vi "CODMn通讯.vi"() -> ()   [LabVIEW 2016, in "斯坦道CODMn.lvlib"]
uses:
  <vilib>/NI/Modbus Library/API/Wrapper/Create TCP Slave.vi
  <vilib>/NI/Modbus Library/API/slave/Modbus Slave.lvclass
  <vilib>/Plasmionique/MB Master/MB_Master/MB_Master.lvclass
  <vilib>/Plasmionique/MB Master/MB Master.lvlib
  <vilib>/Utility/config.llb/NI_LVConfig.lvlib
  <vilib>/NI/Modbus Library/API/Wrapper/API Main.lvlib
panel:
  in  "读取数据":bool
  in  "释放串口":bool
  in  "打开串口":bool
  out "队列中元素数量":i32
  out "元素":cluster{"命令":string}[](array[cluster])
  out "待处理插入数量":i32
  out "读取公式":u16[](array[numeric])
  out "读取参数":u16[](array[numeric])
  out "数据存储":u16[](array[numeric])
  out "温度":bool[](array[boolean])
  out "M输出点":bool[](array[boolean])
  out "ORP、时间":u16[](array[numeric])
  out "测量状态":u16[](array[numeric])
  out "通讯状态":bool
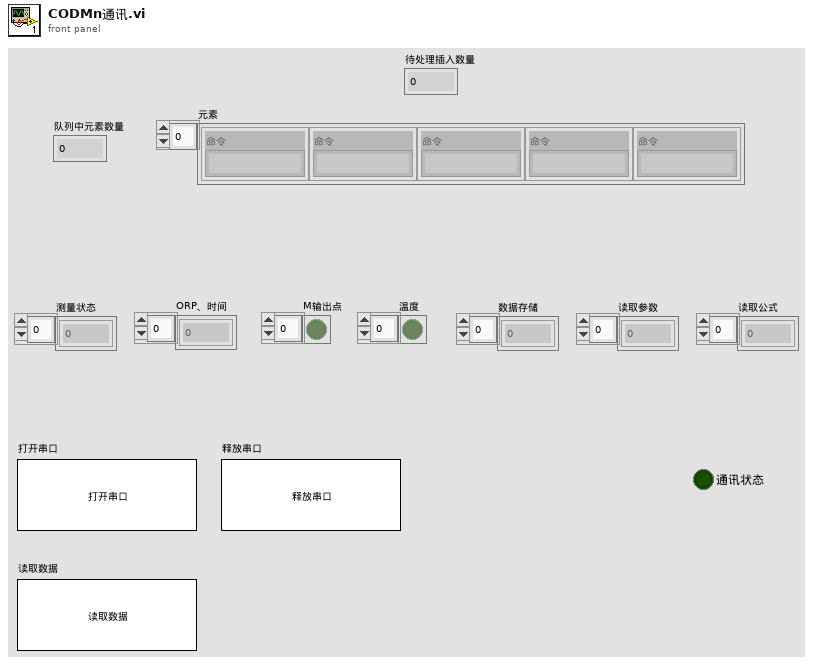
[diagram p1: front panel]
types:
  T1 = cluster{"测量模式":enum16{"水样测量", "标样核查", "零点核查", "跨度核查", "空白测试", "加标回收", "平行样", "校零", "校标"}}
  T2 = cluster{"命令":string, "测量模式":enum16{"水样测量", "标样核查", "零点核查", "跨度核查", "空白测试", "加标回收", "平行样", "校零", "校标"}, "CODMn量程切换":enum32{"H", "L", "AUTO"}}
  T3 = typedef "NI_LVConfig.lvlib/Config Data RefNum.ctl" = refnum<k1>
  T4 = enum16{"空闲", "水样测试", "标样核查", "零点核查", "跨度核查", "空白测试", "平行样测试", "质控样", "空白校准", "标样校准", "加标回收"}
  T5 = enum16{"水样测量", "标样核查", "零点核查", "跨度核查", "空白测试", "加标回收", "平行样", "校零", "校标"}
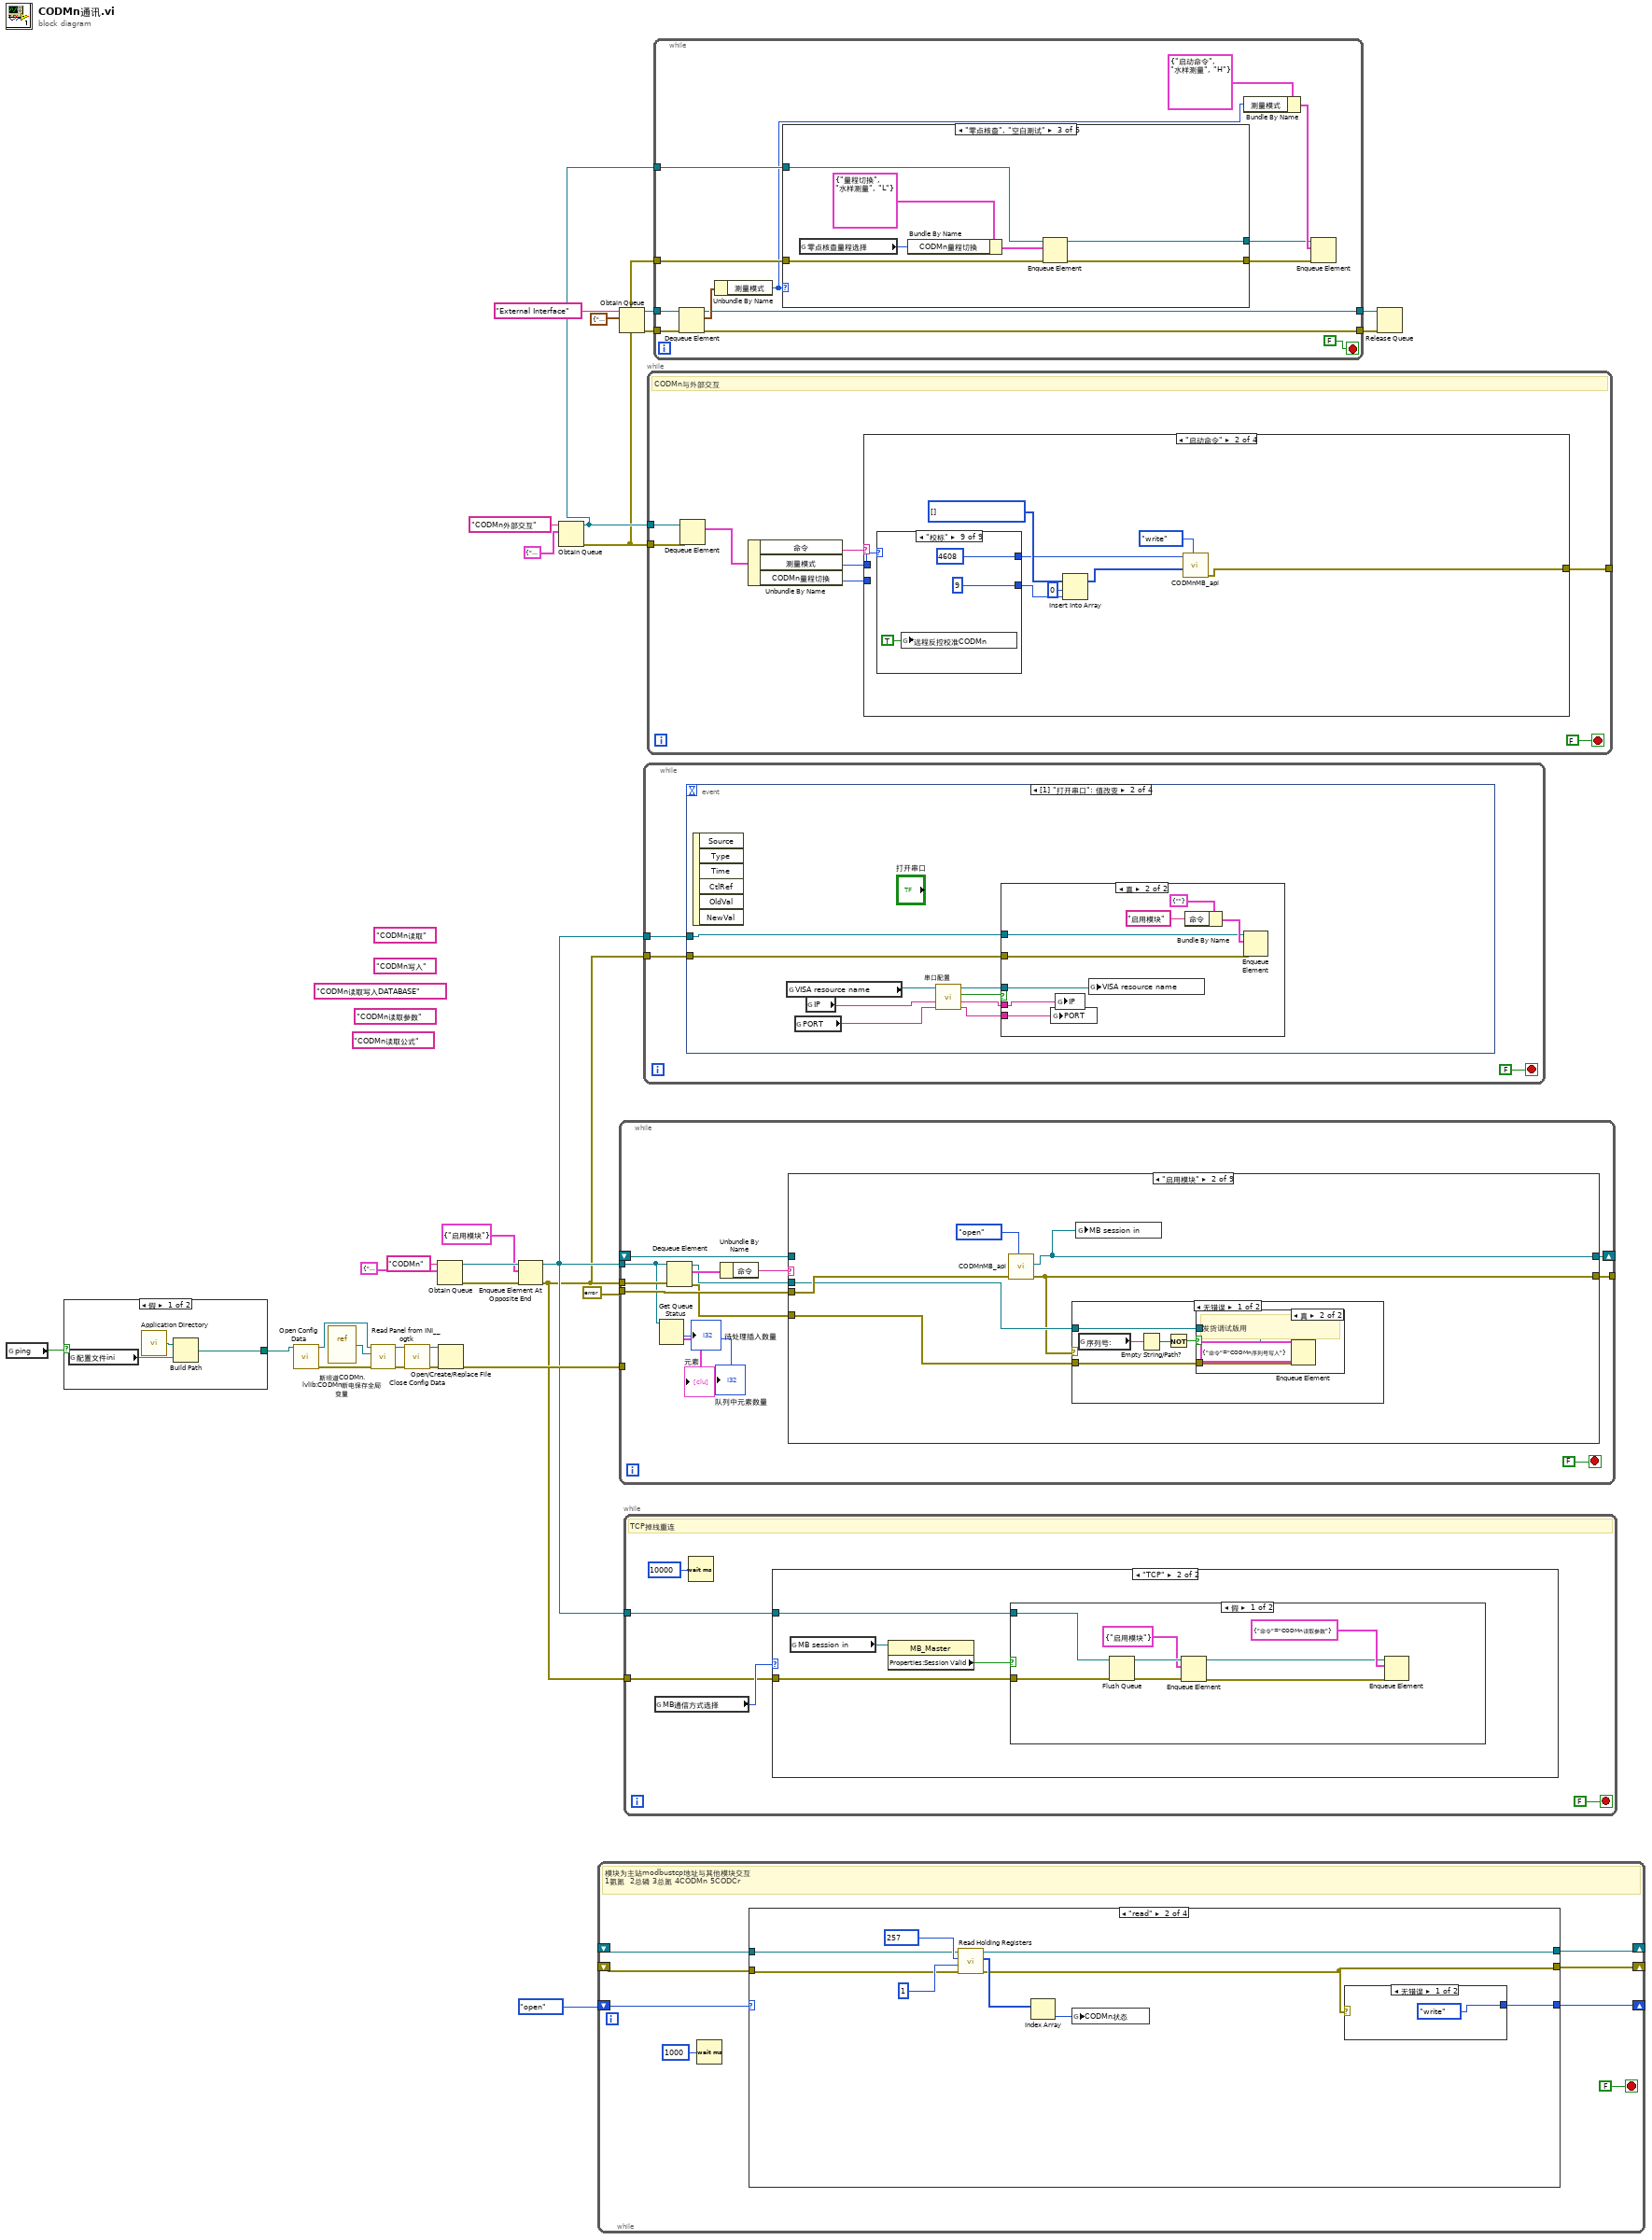
[diagram p0: block diagram]
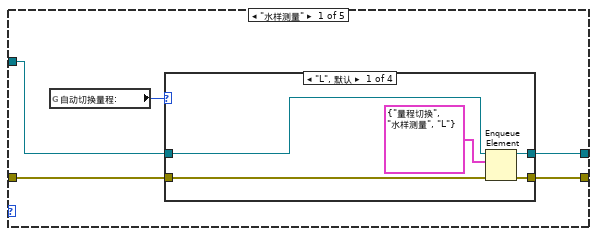
[diagram p2: hidden frame]
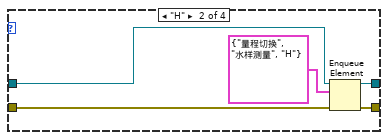
[diagram p3: hidden frame]
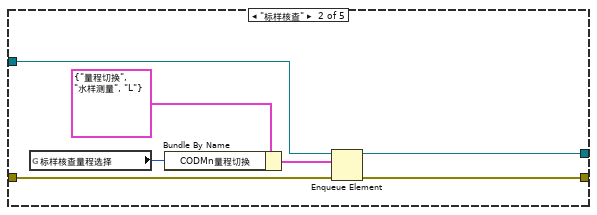
[diagram p6: hidden frame]
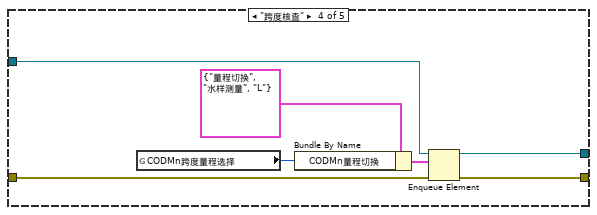
[diagram p7: hidden frame]
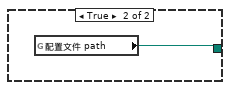
[diagram p9: hidden frame]
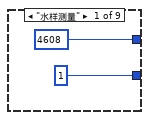
[diagram p11: hidden frame]
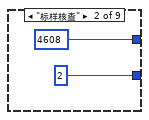
[diagram p12: hidden frame]
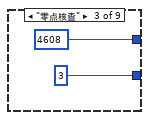
[diagram p13: hidden frame]
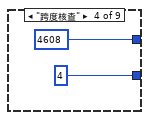
[diagram p14: hidden frame]
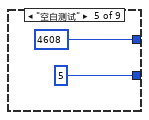
[diagram p15: hidden frame]
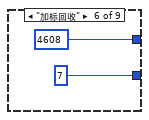
[diagram p16: hidden frame]
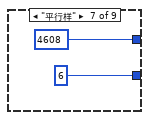
[diagram p17: hidden frame]
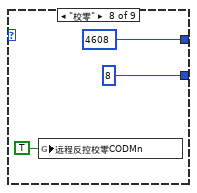
[diagram p18: hidden frame]
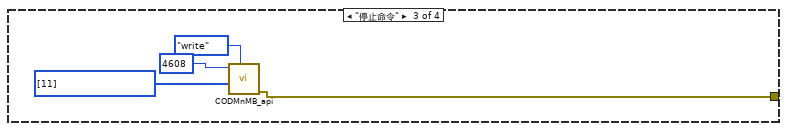
[diagram p19: hidden frame]
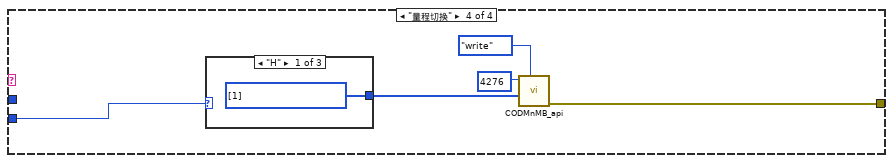
[diagram p20: hidden frame]
diagram:
  (unwired) "CODMn读取公式" ("名称（未命名）")
  (unwired) "CODMn读取写入DATABASE" ("名称（未命名）")
  (unwired) "CODMn读取参数" ("名称（未命名）")
  (unwired) "CODMn读取" ("名称（未命名）")
  (unwired) "CODMn写入" ("名称（未命名）")
  n1 = global read "CODMN外部API.vi" "ping"() -> (w10:bool)
  n2 = case shown="假" w10 {
    tunnel: [w30 w33] -> w9
    frame False {
      n3 = global read "COD内部交互全局.vi" "配置文件ini"() -> (w32:string)
      n4 = call <vilib>:"Application Directory.vi"() -> ("Application Directory"=w31:path)
      n5 = Build Path(base path=w31, name or relative path=w32) -> (appended path=w30:path)
    }
    frame True {
      n6 = global read "CODMN外部API.vi" "配置文件 path"() -> (w33:path)
    }
  }
  n7 = call <vilib>:"Open Config Data.vi"("configuration file path"=w9) -> ("error out"=w20:errorcluster, "refnum"=w23:T3)  [unwired: 8 in, 1 out]
  n8 = vi-ref "斯坦道CODMn.lvlib:CODMn断电保存全局变量.vi"() -> (w22:refnum<vi>)
  n9 = call <userlib>:"Read Panel from INI__ogtk.vi"("error in (no error)"=w20, "VI ref"=w22, "refnum"=w23) -> ("error out"=w19:errorcluster, "refnum out"=w21:T3)  [unwired: 7 in]
  n10 = call <vilib>:"Close Config Data.vi"("error in (no error)"=w19, "refnum"=w21) -> ("error out"=w18:errorcluster, "file path"=w17:path)  [unwired: 8 in]
  n11 = Obtain Queue(name (unnamed)="CODMn" ("名称（未命名）"), element data type=cluster{"命令":string} {"命令"="启用模块"} ("元素")) -> (queue out=w26:refnum<queue>, error out=w25:errorcluster)  [unwired: 3 in, 1 out]
  n12 = Open/Create/Replace File(file path (use dialog)=w17, error in=w18) -> (error out=w16:errorcluster)  [unwired: 4 in, 2 out]
  n13 = Enqueue Element At Opposite End(queue=w26, element=cluster{"命令":string} {"命令"="启用模块"} ("元素"), error in (no error)=w25) -> (queue out=w14:refnum<queue>, error out=w13:errorcluster)  [unwired: 1 in, 1 out]
  n14 = Obtain Queue(name (unnamed)="CODMn外部交互" ("名称（未命名）"), element data type=T2 {"命令"="启动命令", "测量模式"=enum."水样测量", "CODMn量程切换"=enum."AUTO"} ("元素")) -> (queue out=w4:refnum<queue>, error out=w3:errorcluster)  [unwired: 3 in, 1 out]
  n15 = while {
    shift-right: [w39] -> _
    shift-left: _ -> [w41]
    shift-right: [w38] -> _
    shift-left: _ -> [w40]
    shift-right: [w35] -> _
    shift-left: enum16{"open", "read", "write", "close"}."open" -> [w36]
    stop <- FALSE stop-if-true
    # "模块为主站modbustcp地址与其他模块交互\n1氨氮  2总磷 3总氮 4CODMn 5CODCr"
    n16 = Wait (ms)(milliseconds to wait=u32 1000 ("等待时间（毫秒）")) -> ()  [unwired: 1 out]
    n17 = case shown="\"read\"" w36 {
      selector: w36 -> [w50 _ _ _]
      tunnel: w41 -> [w44 w58 w81 w87]
      tunnel: w40 -> [w43 w57 w78 w86]
      tunnel: [w47 w53 w80 w87] -> w39
      tunnel: [w46 w54 w79 w89] -> w38
      tunnel: [w49 w61 w82 enum16{"open", "read", "write", "close"}."open"] -> w35
      frame "open", Default {
        n18 = call-dynamic "Shutdown.vi"("error in"=w43, "Modbus slave in"=w44) -> ("error out"=w42:errorcluster)  [unwired: 9 in]
        n19 = call <vilib>:"Clear Errors.vi"("error in (no error)"=w42) -> ("error out"=w45:errorcluster)  [unwired: 5 in, 1 out]
        n20 = call-poly <vilib>:"Create Modbus Instance.vi"("error in"=w45, "port (502)"=u16 4) -> ("error out"=w46:errorcluster, "TCP slave instance"=w47:refnum<class "Modbus Slave.lvclass">)  [unwired: 8 in]
        n21 = case shown="错误" w46 {
          tunnel: w50 -> [_ w52]
          tunnel: [enum16{"open", "read", "write", "close"}."write" w52] -> w49
          frame No Error {
          }
          frame Error {
          }
        }
      }
      frame "read" {
        n22 = call-dynamic <vilib>:"Read Holding Registers.vi"("error in"=w57, "number of inputs"=u16 1, "starting address"=u16 257, "Modbus slave in"=w58) -> ("error out"=w54:errorcluster, "register values"=w56:u16[], "Modbus slave out"=w53:refnum<class "Modbus Slave.lvclass">)  [unwired: 5 in]
        n23 = Index Array(array=w56) -> (element=w55:u16)  [unwired: 1 in]
        n24 = global write "CODMN外部API.vi" "CODMn状态"(w55) -> ()
        n25 = case shown="无错误" w54 {
          tunnel: [enum16{"open", "read", "write", "close"}."write" enum16{"open", "read", "write", "close"}."close"] -> w61
          frame No Error {
          }
          frame Error {
          }
        }
      }
      frame "write" {
        n26 = global read "COD测量模式全局.vi" "CODMn工作状态"() -> (w68:T4)
        n27 = global read "COD浓度全局变量.vi" "COD浓度（mg/L)"() -> (w70:dbl)
        n28 = global read "COD测量模式全局.vi" "加标回收启动时间"() -> (w73:timestamp)
        n29 = global read "COD测量模式全局.vi" "水样启动时间"() -> (w75:timestamp)
        n30 = global read "运行时序全局变量.vi" "多列列表框"() -> (w72:i32)
        n31 = Build Array(w75) -> (w74:timestamp[])
        n32 = Build Array(w70) -> (w69:dbl[])
        n33 = Build Array(w73) -> (w66:timestamp[])
        n34 = call "浮点转CDAB整形cod.vi"("浮点数"=w69) -> ("CDAB整形输出"=w71:u16[])  [unwired: 10 in]
        n35 = call "DateToHex.vi"("DATE"=w74) -> ("数组"=w77:u16[])  [unwired: 10 in]
        n36 = call "DateToHex.vi"("DATE"=w66) -> ("数组"=w76:u16[])  [unwired: 10 in]
        n37 = Insert Into Array(array=u16[] [] ("values"), new element #1=w68, new element #2=w71, new element #3=w72, new element #4=w76, new element #5=w77) -> (w65:u16[])  [unwired: 1 in]
        n38 = call-dynamic "Write Multiple Holding Registers.vi"("error in"=w78, "registers to write"=w65, "starting address"=u16 0, "Modbus slave in"=w81) -> ("error out"=w79:errorcluster, "Modbus slave out"=w80:refnum<class "Modbus Slave.lvclass">)  [unwired: 6 in]
        n39 = case shown="无错误" w79 {
          tunnel: [enum16{"open", "read", "write", "close"}."read" enum16{"open", "read", "write", "close"}."close"] -> w82
          frame No Error {
          }
          frame Error {
          }
        }
      }
      frame "close" {
        n40 = call-dynamic "Shutdown.vi"("error in"=w86, "Modbus slave in"=w87) -> ("error out"=w85:errorcluster)  [unwired: 9 in]
        n41 = call <vilib>:"Clear Errors.vi"("error in (no error)"=w85) -> ("error out"=w89:errorcluster)  [unwired: 5 in, 1 out]
      }
    }
  }
  n42 = while {
    tunnel: w14 -> [w95]
    tunnel: w13 -> [w102]
    tunnel: [w96] -> _
    shift-right: [w99] -> _
    shift-left: _ -> [w98]
    tunnel: errorcluster {"status"=FALSE, "code"=0, "source"=""} ("error out") -> [w97]
    tunnel: w16 -> [_]
    stop <- FALSE stop-if-true
    n43 = Get Queue Status(queue=w95) -> (# pending insert=→"待处理插入数量":i32, # elements in queue=→"队列中元素数量":i32, elements=→"元素":cluster{"命令":string}[])  [unwired: 2 in, 5 out]
    n44 = Dequeue Element(queue=w95, error in (no error)=w102) -> (queue out=w91:refnum<queue>, element=w101:cluster{"命令":string}, error out=w90:errorcluster)  [unwired: 1 in, 1 out]
    n45 = Unbundle By Name(w101) -> ("命令"=w100:string)
    n46 = case shown="\"启用模块\"" w100 {
      tunnel: [w105 w109 w120 w128 w160 w169 w186 w193 w200] -> w99
      tunnel: [w104 w106 w121 w125 w158 w168 w185 w192 w199] -> w96
      tunnel: w98 -> [w105 _ _ w152 w164 w178 w189 w197 w203]
      tunnel: w97 -> [w104 w110 w122 w151 w161 w177 w188 w196 w201]
      tunnel: w91 -> [_ w108 _ _ _ _ _ _ _]
      tunnel: w90 -> [_ w107 _ _ _ _ _ _ _]
      frame Default {
      }
      frame "启用模块" {
        n47 = call "CODMnMB_api.vi"("STEP"=enum16{"open", "read", "write", "close"}."open", "Error in"=w110) -> ("error out"=w106:errorcluster, "MB session out"=w109:refnum<class "MB_Master.lvclass">)  [unwired: 7 in, 1 out]
        n48 = case shown="无错误" w106 {
          tunnel: w108 -> [w116 _]
          tunnel: w107 -> [w115 _]
          frame No Error {
            n49 = global read "COD内部交互全局.vi" "序列号:"() -> (w114:string)
            n50 = Empty String/Path?(string/path=w114) -> (empty?=w113:bool)
            n51 = Not(x=w113) -> (.not. x?=w112:bool)
            n52 = case shown="真" w112 {
              tunnel: w116 -> [_ w119]
              tunnel: w115 -> [_ w118]
              frame False {
              }
              frame True {
                # "发货调试版用"
                n53 = Enqueue Element(queue=w119, element=cluster{"命令":string} {"命令"="CODMn序列号写入"} ("元素"), error in (no error)=w118) -> ()  [unwired: 1 in, 3 out]
              }
            }
          }
          frame Error {
          }
        }
        n54 = global write "COD浓度全局变量.vi" "MB session in"(w109) -> ()
      }
      frame "停用模块" {
        n55 = call "CODMnMB_api.vi"("STEP"=enum16{"open", "read", "write", "close"}."close", "Error in"=w122) -> ("error out"=w121:errorcluster, "MB session out"=w120:refnum<class "MB_Master.lvclass">)  [unwired: 7 in, 1 out]
      }
      frame "CODMn读取" {
        n56 = call <vilib>:"Read Holding Registers.vi"("error in (no error)"=w151, "quantity"=u16 50 ("number of holding registers"), "starting address"=u16 4224, "MB session in"=w152) -> ("error out"=w142:errorcluster, "Registers"=w148:u16[], "MB session out"=w143:refnum<class "MB_Master.lvclass">)  [unwired: 5 in]
        n57 = case shown="无错误" w142 {
          tunnel: w148 -> [w157 _]
          frame No Error {
            n58 = global write "COD内部交互全局.vi" "测量状态"(w157) -> ()
            "测量状态" <- w157
          }
          frame Error {
          }
        }
        n59 = call <vilib>:"Read Holding Registers.vi"("error in (no error)"=w142, "quantity"=u16 10, "starting address"=u16 4101, "MB session in"=w143) -> ("error out"=w138:errorcluster, "Registers"=w141:u16[], "MB session out"=w140:refnum<class "MB_Master.lvclass">)  [unwired: 5 in]
        n60 = case shown="无错误" w138 {
          tunnel: w141 -> [w156 _]
          frame No Error {
            n61 = global write "COD内部交互全局.vi" "ORP、时间"(w156) -> ()
            "ORP、时间" <- w156
          }
          frame Error {
          }
        }
        n62 = call <vilib>:"Read Coils.vi"("error in (no error)"=w138, "quantity"=u16 11, "starting address"=u16 137, "MB session in"=w140) -> ("error out"=w136:errorcluster, "Coils"=w137:bool[], "MB session out"=w139:refnum<class "MB_Master.lvclass">)  [unwired: 5 in]
        n63 = case shown="无错误" w136 {
          tunnel: w137 -> [w155 _]
          frame No Error {
            n64 = global write "COD内部交互全局.vi" "M输出点"(w155) -> ()
            "M输出点" <- w155
          }
          frame Error {
          }
        }
        n65 = call <vilib>:"Read Coils.vi"("error in (no error)"=w136, "quantity"=u16 1, "starting address"=u16 400, "MB session in"=w139) -> ("error out"=w129:errorcluster, "Coils"=w133:bool[], "MB session out"=w130:refnum<class "MB_Master.lvclass">)  [unwired: 5 in]
        n66 = case shown="无错误" w129 {
          tunnel: w133 -> [w154 _]
          frame No Error {
            n67 = global write "COD内部交互全局.vi" "温度"(w154) -> ()
            "温度" <- w154
          }
          frame Error {
          }
        }
        n68 = call <vilib>:"Read Coils.vi"("error in (no error)"=w129, "quantity"=u16 20, "starting address"=u16 500, "MB session in"=w130) -> ("error out"=w125:errorcluster, "Coils"=w124:bool[], "MB session out"=w128:refnum<class "MB_Master.lvclass">)  [unwired: 5 in]
        n69 = case shown="无错误" w125 {
          tunnel: w124 -> [w153 _]
          frame No Error {
            n70 = global write "COD内部交互全局.vi" "报警点位"(w153) -> ()
          }
          frame Error {
          }
        }
        n71 = Unbundle By Name(w125) -> ("status"=w132:bool)
        n72 = Not(x=w132) -> (.not. x?=w131:bool)
        "通讯状态" <- w131
        n73 = global write "COD内部交互全局.vi" "通讯状态"(w131) -> ()
      }
      frame "CODMn读取写入DATABASE" {
        n74 = call <vilib>:"Read Holding Registers.vi"("error in (no error)"=w161, "quantity"=u16 10 ("number of holding registers"), "starting address"=u16 4101, "MB session in"=w164) -> ("error out"=w158:errorcluster, "Registers"=w159:u16[], "MB session out"=w160:refnum<class "MB_Master.lvclass">)  [unwired: 5 in]
        n75 = case shown="无错误" w158 {
          tunnel: w159 -> [w166 _]
          frame No Error {
            n76 = global write "COD内部交互全局.vi" "数据存储"(w166) -> ()
            n77 = global write "COD内部交互全局.vi" "读取写入data"(TRUE ("读取参数显示")) -> ()
            "数据存储" <- w166
          }
          frame Error {
          }
        }
      }
      frame "CODMn读取参数" {
        n78 = call <vilib>:"Read Holding Registers.vi"("error in (no error)"=w177, "quantity"=u16 35 ("number of holding registers"), "starting address"=u16 4272, "MB session in"=w178) -> ("error out"=w172:errorcluster, "Registers"=w174:u16[], "MB session out"=w173:refnum<class "MB_Master.lvclass">)  [unwired: 5 in]
        n79 = case shown="无错误" w172 {
          tunnel: w174 -> [w182 _]
          frame No Error {
            n80 = global write "COD内部交互全局.vi" "读取参数"(w182) -> ()
            n81 = global write "COD内部交互全局.vi" "读取参数显示"(TRUE ("读取参数显示")) -> ()
            "读取参数" <- w182
          }
          frame Error {
          }
        }
        n82 = call <vilib>:"Read Holding Registers.vi"("error in (no error)"=w172, "quantity"=u16 4, "starting address"=u16 5596, "MB session in"=w173) -> ("error out"=w168:errorcluster, "Registers"=w167:u16[], "MB session out"=w169:refnum<class "MB_Master.lvclass">)  [unwired: 5 in]
        n83 = case shown="无错误" w168 {
          tunnel: w167 -> [w180 _]
          frame No Error {
            n84 = global write "COD内部交互全局.vi" "读取浮台参数"(w180) -> ()
            n85 = global write "COD内部交互全局.vi" "读取浮台参数显示"(TRUE ("读取参数显示")) -> ()
          }
          frame Error {
          }
        }
      }
      frame "CODMn读取公式" {
        n86 = call <vilib>:"Read Holding Registers.vi"("error in (no error)"=w188, "quantity"=u16 94 ("number of holding registers"), "starting address"=u16 4616, "MB session in"=w189) -> ("error out"=w185:errorcluster, "Registers"=w187:u16[], "MB session out"=w186:refnum<class "MB_Master.lvclass">)  [unwired: 5 in]
        n87 = case shown="无错误" w185 {
          tunnel: w187 -> [w191 _]
          frame No Error {
            n88 = global write "COD内部交互全局.vi" "读取公式"(w191) -> ()
            n89 = global write "COD内部交互全局.vi" "读取公式显示"(TRUE ("读取参数显示")) -> ()
            "读取公式" <- w191
          }
          frame Error {
          }
        }
      }
      frame "CODMn序列号写入" {
        n90 = global read "COD内部交互全局.vi" "序列号:"() -> (w195:string)
        n91 = call "StringToHex.vi"("STRING"=w195) -> ("数组"=w194:u16[])  [unwired: 10 in]
        n92 = call <vilib>:"Write Multiple Registers.vi"("error in (no error)"=w196, "values"=w194, "starting address"=u16 4298, "MB session in"=w197) -> ("error out"=w192:errorcluster, "MB session out"=w193:refnum<class "MB_Master.lvclass">)  [unwired: 6 in]
      }
      frame "CODMn程序更新" {
        n93 = call <vilib>:"Write Multiple Registers.vi"("error in (no error)"=w201, "values"=u16[] [0], "starting address"=u16 4296, "MB session in"=w203) -> ("error out"=w199:errorcluster, "MB session out"=w200:refnum<class "MB_Master.lvclass">)  [unwired: 6 in]
      }
    }
  }
  n94 = Obtain Queue(name (unnamed)="External Interface" ("名称（未命名）"), element data type=T1 {"测量模式"=enum."水样测量"} ("启动测量模式")) -> (queue out=w6:refnum<queue>, error out=w5:errorcluster)  [unwired: 3 in, 1 out]
  n95 = while "While循环" {
    tunnel: w14 -> [w206]
    tunnel: w13 -> [w205]
    stop <- FALSE stop-if-true
    # "TCP掉线重连"
    n96 = global read "CODMn断电保存全局变量.vi" "MB通信方式选择"() -> (w207:enum16{"串口", "TCP"})
    n97 = Wait (ms)(milliseconds to wait=u32 10000 ("等待时间（毫秒）")) -> ()  [unwired: 1 out]
    n98 = case shown="\"TCP\"" w207 {
      tunnel: w206 -> [_ w211]
      tunnel: w205 -> [_ w210]
      frame "串口", Default {
      }
      frame "TCP" {
        n99 = global read "COD浓度全局变量.vi" "MB session in"() -> (w213:refnum<class "MB_Master.lvclass">)
        n100 = property class="MB_Master"(reference=w213) -> ("Properties:Session Valid"=w212:bool)  [unwired: 1 in, 2 out]
        n101 = case shown="假" w212 {
          tunnel: w211 -> [w218 _]
          tunnel: w210 -> [w217 _]
          frame False {
            n102 = Flush Queue(queue=w218, error in (no error)=w217) -> (queue out=w221:refnum<queue>, error out=w220:errorcluster)  [unwired: 1 out]
            n103 = Enqueue Element(queue=w221, element=cluster{"命令":string} {"命令"="启用模块"} ("元素"), error in (no error)=w220) -> (queue out=w215:refnum<queue>, error out=w214:errorcluster)  [unwired: 1 in, 1 out]
            n104 = Enqueue Element(queue=w215, element=cluster{"命令":string} {"命令"="CODMn读取参数"} ("元素"), error in (no error)=w214) -> ()  [unwired: 1 in, 3 out]
          }
          frame True {
          }
        }
      }
    }
  }
  n105 = while {
    tunnel: w14 -> [w223]
    tunnel: w13 -> [w222]
    stop <- FALSE stop-if-true
    n106 = event shown="[1] \"打开串口\": 值改变" {
      selector: _ -> [_ _ _ _]
      dyn-events: _ -> [_ _ _ _]
      timeout: _ -> [_ _ _ _]
      tunnel: w223 -> [_ w230 w244 w246]
      tunnel: w222 -> [_ w229 w243 w245]
      event Timeout {
        n107 = event-data() -> ()  [unwired: 1 in, 3 out]
      }
      event "打开串口": Value Change {
        n108 = event-data() -> ()  [unwired: 1 in, 6 out]
        n109 = global read "CODMn断电保存全局变量.vi" "VISA resource name"() -> (w233:refnum<visa-resource-name>)
        n110 = global read "CODMn断电保存全局变量.vi" "PORT"() -> (w225:string)
        n111 = global read "CODMn断电保存全局变量.vi" "IP"() -> (w226:string)
        n112 = call "串口配置.vi"("PORT"=w225, "IP"=w226, "请选择串口:"=w233) -> ("PORT 2"=w227:string, "IP 2"=w228:string, "确认 2"=w231:bool, "VISA资源名称 2"=w232:refnum<visa-resource-name>)  [unwired: 4 in, 1 out]
        n113 = case shown="真" w231 {
          tunnel: w232 -> [_ w241]
          tunnel: w230 -> [_ w237]
          tunnel: w229 -> [_ w236]
          tunnel: w228 -> [_ w235]
          tunnel: w227 -> [_ w234]
          frame False {
          }
          frame True {
            n114 = global write "CODMn断电保存全局变量.vi" "PORT"(w234) -> ()
            n115 = global write "CODMn断电保存全局变量.vi" "IP"(w235) -> ()
            n116 = global write "CODMn断电保存全局变量.vi" "VISA resource name"(w241) -> ()
            n117 = Bundle By Name(cluster=cluster{"命令":string} {"命令"=""} ("元素"), "命令"="启用模块" ("名称（未命名）")) -> (w238:cluster{"命令":string})
            n118 = Enqueue Element(queue=w237, element=w238, error in (no error)=w236) -> ()  [unwired: 1 in, 3 out]
          }
        }
      }
      event "释放串口": Value Change {
        n119 = event-data() -> ()  [unwired: 1 in, 6 out]
        n120 = Enqueue Element(queue=w244, element=cluster{"命令":string} {"命令"="停用模块"} ("元素"), error in (no error)=w243) -> ()  [unwired: 1 in, 3 out]
      }
      event "读取数据": Value Change {
        n121 = event-data() -> ()  [unwired: 1 in, 6 out]
        n122 = Enqueue Element(queue=w246, element=cluster{"命令":string} {"命令"="CODMn读取"} ("元素"), error in (no error)=w245) -> ()  [unwired: 1 in, 3 out]
      }
    }
  }
  n123 = while {
    tunnel: w4 -> [w253]
    tunnel: w3 -> [w252]
    tunnel: [w248] -> _
    stop <- FALSE stop-if-true
    # "CODMn与外部交互"
    n124 = Dequeue Element(queue=w253, error in (no error)=w252) -> (element=w254:T2)  [unwired: 1 in, 3 out]
    n125 = Unbundle By Name(w254) -> ("命令"=w251:string, "测量模式"=w250:T5, "CODMn量程切换"=w249:enum32{"H", "L", "AUTO"})
    n126 = case shown="\"启动命令\"" w251 {
      tunnel: w250 -> [_ w257 _ _]
      tunnel: w249 -> [_ _ _ w289]
      tunnel: [_ w256 w284 w288] -> w248
      frame "假", Default {
      }
      frame "启动命令" {
        n127 = case shown="\"校标\"" w257 {
          tunnel: [u16 4608 ("address") u16 4608 ("address") u16 4608 ("address") u16 4608 ("address") u16 4608 ("address") u16 4608 ("address") u16 4608 ("address") u16 4608 ("address") u16 4608 ("address")] -> w259
          tunnel: [u16 1 ("address") u16 2 ("address") u16 3 ("address") u16 4 ("address") u16 5 ("address") u16 7 ("address") u16 6 ("address") u16 8 ("address") u16 9 ("address")] -> w263
          frame "水样测量" {
          }
          frame "标样核查" {
          }
          frame "零点核查" {
          }
          frame "跨度核查" {
          }
          frame "空白测试" {
          }
          frame "加标回收" {
          }
          frame "平行样" {
          }
          frame "校零" {
            n128 = global write "CODMN外部API.vi" "远程反控校零CODMn"(TRUE ("远程反控校准CODMn")) -> ()
          }
          frame "校标" {
            n129 = global write "CODMN外部API.vi" "远程反控校准CODMn"(TRUE ("远程反控校准CODMn")) -> ()
          }
        }
        n130 = Insert Into Array(array=u16[] [] ("values"), index=0 ("索引"), new element=w263) -> (w258:u16[])
        n131 = call "CODMnMB_api.vi"("STEP"=enum16{"open", "read", "write", "close"}."write", "values"=w258, "starting address"=w259) -> ("error out"=w256:errorcluster)  [unwired: 6 in, 2 out]
      }
      frame "停止命令" {
        n132 = call "CODMnMB_api.vi"("STEP"=enum16{"open", "read", "write", "close"}."write", "values"=u16[] [11], "starting address"=u16 4608) -> ("error out"=w284:errorcluster)  [unwired: 6 in, 2 out]
      }
      frame "量程切换" {
        n133 = case shown="\"H\"" w289 {
          tunnel: [u16[] [1] ("values") u16[] [0] ("values") _] -> w292
          frame "H" {
          }
          frame "L" {
          }
          frame "AUTO", Default {
          }
        }
        n134 = call "CODMnMB_api.vi"("STEP"=enum16{"open", "read", "write", "close"}."write", "values"=w292, "starting address"=u16 4276) -> ("error out"=w288:errorcluster)  [unwired: 6 in, 2 out]
      }
    }
  }
  n135 = while {
    tunnel: w6 -> [w307]
    tunnel: w5 -> [w306]
    tunnel: w4 -> [w303]
    tunnel: w3 -> [w302]
    tunnel: [w296] -> w2
    tunnel: [w295] -> w1
    stop <- FALSE stop-if-true
    n136 = Dequeue Element(queue=w307, error in (no error)=w306) -> (queue out=w296:refnum<queue>, element=w304:T1, error out=w295:errorcluster)  [unwired: 1 in, 1 out]
    n137 = Unbundle By Name(w304) -> ("测量模式"=w299:T5)
    n138 = case "条件结构" shown="\"零点核查\", \"空白测试\"" w299 {
      tunnel: w303 -> [w311 w330 w337 w344 w349]
      tunnel: w302 -> [w309 w329 w336 w343 w348]
      tunnel: [w310 w328 w335 w342 w349] -> w298
      tunnel: [w308 w327 w334 w341 w348] -> w297
      frame "水样测量" {
        n139 = global read "CODMn断电保存全局变量.vi" "自动切换量程:"() -> (w312:enum16{"L", "H", "自动切换测一次", "自动切换测两次"})
        n140 = case shown="\"L\", 默认" w312 {
          tunnel: w311 -> [w316 w322 w323 w326]
          tunnel: [w314 w321 w323 w326] -> w310
          tunnel: w309 -> [w315 w320 w324 w325]
          tunnel: [w313 w319 w324 w325] -> w308
          frame "L", Default {
            n141 = Enqueue Element(queue=w316, element=T2 {"命令"="量程切换", "测量模式"=enum."水样测量", "CODMn量程切换"=enum."L"} ("元素"), error in (no error)=w315) -> (queue out=w314:refnum<queue>, error out=w313:errorcluster)  [unwired: 1 in, 1 out]
          }
          frame "H" {
            n142 = Enqueue Element(queue=w322, element=T2 {"命令"="量程切换", "测量模式"=enum."水样测量", "CODMn量程切换"=enum."H"} ("元素"), error in (no error)=w320) -> (queue out=w321:refnum<queue>, error out=w319:errorcluster)  [unwired: 1 in, 1 out]
          }
          frame "自动切换测一次" {
          }
          frame "自动切换测两次" {
          }
        }
      }
      frame "标样核查" {
        n143 = global read "CODMn断电保存全局变量.vi" "标样核查量程选择"() -> (w332:enum32{"H", "L", "AUTO"})
        n144 = Bundle By Name(cluster=T2 {"命令"="量程切换", "测量模式"=enum."水样测量", "CODMn量程切换"=enum."L"} ("元素"), "CODMn量程切换"=w332) -> (w333:T2)
        n145 = Enqueue Element(queue=w330, element=w333, error in (no error)=w329) -> (queue out=w328:refnum<queue>, error out=w327:errorcluster)  [unwired: 1 in, 1 out]
      }
      frame "零点核查", "空白测试" {
        n146 = global read "CODMn断电保存全局变量.vi" "零点核查量程选择"() -> (w339:enum32{"H", "L", "AUTO"})
        n147 = Bundle By Name(cluster=T2 {"命令"="量程切换", "测量模式"=enum."水样测量", "CODMn量程切换"=enum."L"} ("元素"), "CODMn量程切换"=w339) -> (w338:T2)
        n148 = Enqueue Element(queue=w337, element=w338, error in (no error)=w336) -> (queue out=w335:refnum<queue>, error out=w334:errorcluster)  [unwired: 1 in, 1 out]
      }
      frame "跨度核查" {
        n149 = global read "CODMn断电保存全局变量.vi" "CODMn跨度量程选择"() -> (w346:enum32{"H", "L", "AUTO"})
        n150 = Bundle By Name(cluster=T2 {"命令"="量程切换", "测量模式"=enum."水样测量", "CODMn量程切换"=enum."L"} ("元素"), "CODMn量程切换"=w346) -> (w345:T2)
        n151 = Enqueue Element(queue=w344, element=w345, error in (no error)=w343) -> (queue out=w342:refnum<queue>, error out=w341:errorcluster)  [unwired: 1 in, 1 out]
      }
      frame Default {
        # "不切换量程"
      }
    }
    n152 = Bundle By Name(cluster=T2 {"命令"="启动命令", "测量模式"=enum."水样测量", "CODMn量程切换"=enum."H"} ("元素"), "测量模式"=w299) -> (w300:T2)
    n153 = Enqueue Element(queue=w298, element=w300, error in (no error)=w297) -> ()  [unwired: 1 in, 3 out]
  }
  n154 = Release Queue(queue=w2, error in (no error)=w1) -> ()  [unwired: 1 in, 3 out]
